vi "4 QuadEncoder PositionVelocity.vi"(0 "Quad Encoders":T1={"Encoder 0 Ch A"="Chassis1/Mod4/DI0", "Encoder 0 Ch B"="Chassis1/Mod4/DI1", "Encoder 1 Ch A"="Chassis1/Mod4/DI2", "Encoder 1 Ch B"="Chassis1/Mod4/DI3", "Encoder 2 Ch A"="Chassis1/Mod4/DI4", "Encoder 2 Ch B"="Chassis1/Mod4/DI5", "Encoder 3 Ch A"="Chassis1/Mod4/DI6", "Encoder 3 Ch B"="Chassis1/Mod4/DI7"}, 2 "Encoder Interval (uSec)":u32=1000, 4 "Position Reset":bool) -> (7 "Encoder Packets":u64[](array[numeric]))   [LabVIEW 2010]
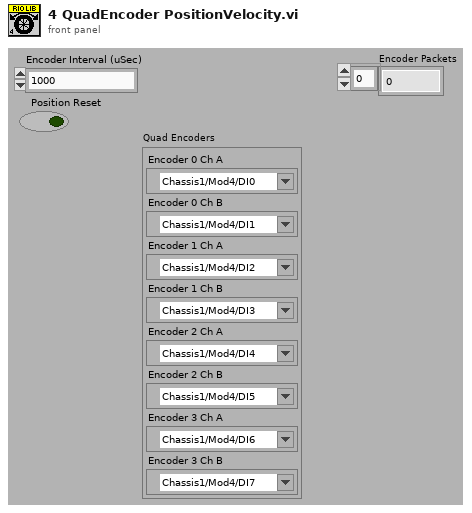
[diagram p1: front panel]
types:
  T1 = cluster{"Encoder 0 Ch A":refnum<k21>, "Encoder 0 Ch B":refnum<k21>, "Encoder 1 Ch A":refnum<k21>, "Encoder 1 Ch B":refnum<k21>, "Encoder 2 Ch A":refnum<k21>, "Encoder 2 Ch B":refnum<k21>, "Encoder 3 Ch A":refnum<k21>, "Encoder 3 Ch B":refnum<k21>}
  T2 = cluster{"Encoder 0 Ch A":refnum<k21>, "Encoder 0 Ch B":refnum<k21>}
  T3 = cluster{"Encoder 1 Ch A":refnum<k21>, "Encoder 1 Ch B":refnum<k21>}
  T4 = cluster{"Encoder 2 Ch A":refnum<k21>, "Encoder 2 Ch B":refnum<k21>}
  T5 = cluster{"Encoder 3 Ch A":refnum<k21>, "Encoder 3 Ch B":refnum<k21>}
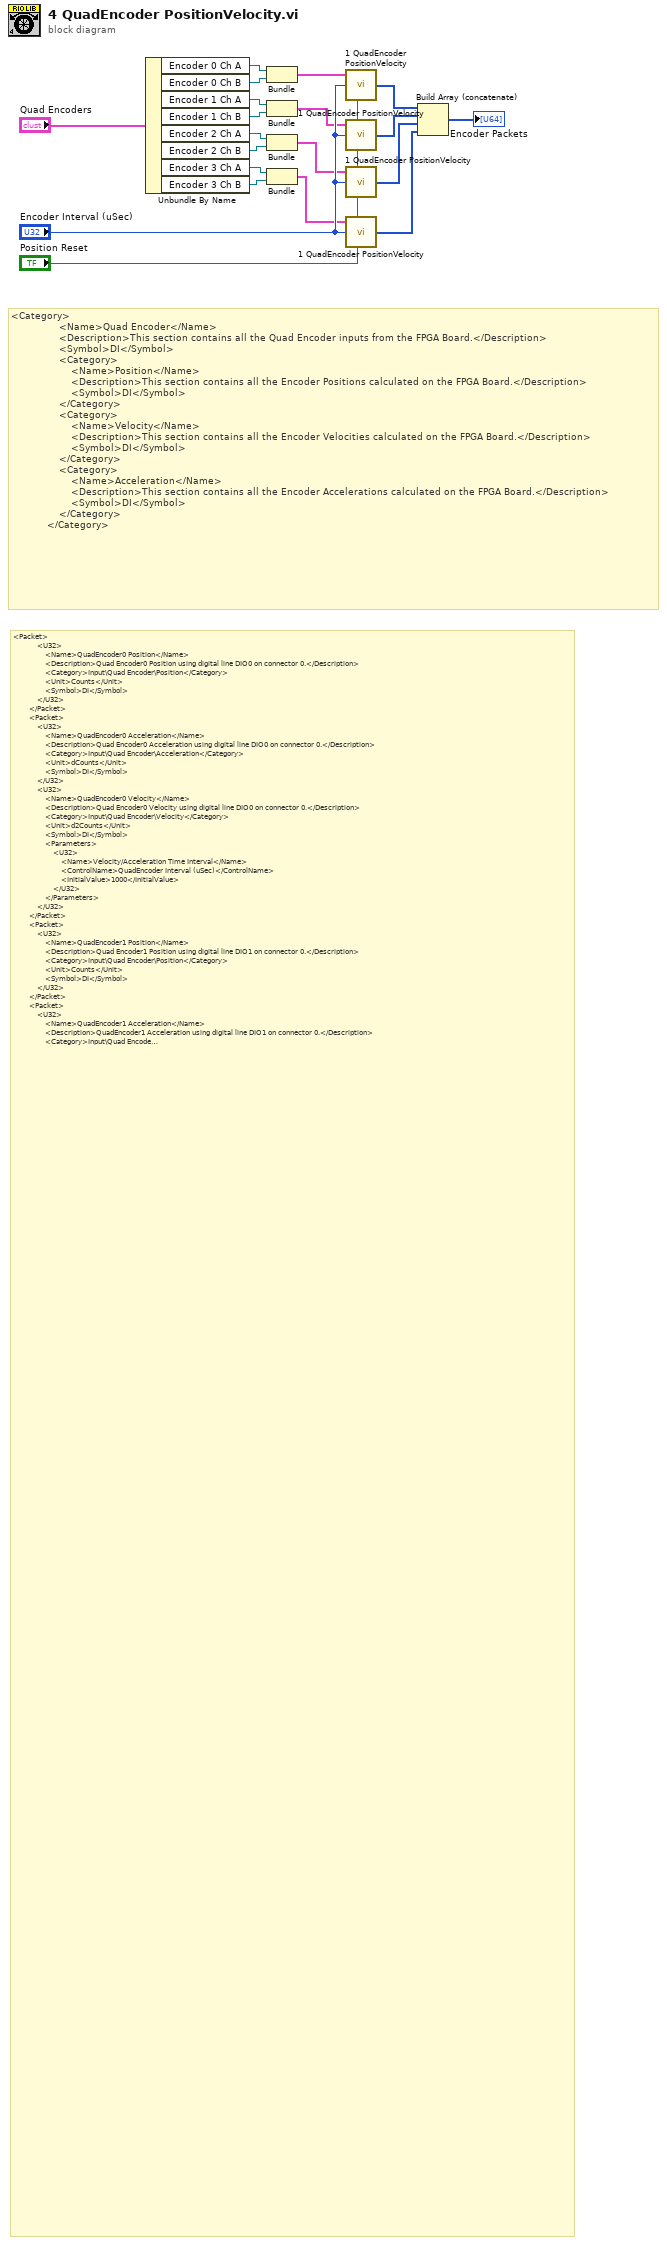
[diagram p0: block diagram]
diagram:
  # "<Category>\n                <Name>Quad Encoder</Name>\n                <Description>This section contains all the Quad Encoder inputs from the FPGA Board.</Description>\n                <Symbol>DI</Symbol>\n                <Category>\n                    <Name>Position</Name>\n                    <Description>This section contains all the Encoder Positions calculated on the FPGA Board.</Description>\n                    <Symbol>DI</Symbol>\n                </Category>\n                <Category>\n                    <Name>Velocity</Name>\n                    <Description>This section contains all the Encoder Velocities calculated on the FPGA Board.</Description>\n                    <Symbol>DI</Symbol>\n                </Category>\n                <Category>\n                    <Name>Acceleration</Name>\n                    <Description>This section contains all the Encoder Accelerations calculated on the FPGA Board.</Description>\n                    <Symbol>DI</Symbol>\n                </Category>\n            </Category>"
  # "<Packet>\n            <U32>\n                <Name>QuadEncoder0 Position</Name>\n                <Description>Quad Encoder0 Position using digital line DIO0 on connector 0.</Description>\n                <Category>Input\\Quad Encoder\\Position</Category>\n                <Unit>Counts</Unit>\n                <Symbol>DI</Symbol>\n            </U32>\n        </Packet>\n        <Packet>\n            <U32>\n                <Name>QuadEncoder0 Acceleration</Name>\n                <Description>Quad Encoder0 Acceleration using digital line DIO0 on connector 0.</Description>\n                <Category>Input\\Quad Encoder\\Acceleration</Category>\n                <Unit>dCounts</Unit>\n                <Symbol>DI</Symbol>\n            </U32>\n            <U32>\n                <Name>QuadEncoder0 Velocity</Name>\n                <Description>Quad Encoder0 Velocity using digital line DIO0 on connector 0.</Description>\n                <Category>Input\\Quad Encoder\\Velocity</Category>\n                <Unit>d2Counts</Unit>\n                <Symbol>DI</Symbol>\n                <Parameters>\n                    <U32>\n                        <Name>Velocity/Acceleration Time Interval</Name>\n                        <ControlName>QuadEncoder Interval (uSec)</ControlName>\n                        <InitialValue>1000</InitialValue>\n                    </U32>\n                </Parameters>\n            </U32>\n        </Packet>\n        <Packet>\n            <U32>\n                <Name>QuadEncoder1 Position</Name>\n                <Description>Quad Encoder1 Position using digital line DIO1 on connector 0.</Description>\n                <Category>Input\\Quad Encoder\\Position</Category>\n                <Unit>Counts</Unit>\n                <Symbol>DI</Symbol>\n            </U32>\n        </Packet>\n        <Packet>\n            <U32>\n                <Name>QuadEncoder1 Acceleration</Name>\n                <Description>QuadEncoder1 Acceleration using digital line DIO1 on connector 0.</Description>\n                <Category>Input\\Quad Encoder\\Acceleration</Category>\n                <Unit>dCounts</Unit>\n                <Symbol>DI</Symbol>\n            </U32>\n            <U32>\n                <Name>QuadEncoder1 Velocity</Name>\n                <Description>QuadEncoder1 Velocity using digital line DIO1 on connector 0.</Description>\n                <Category>Input\\Quad Encoder\\Velocity</Category>\n                <Unit>d2Counts</Unit>\n                <Symbol>DI</Symbol>\n            </U32>\n        </Packet>\n        <Packet>\n            <U32>\n                <Name>QuadEncoder2 Position</Name>\n                <Description>Quad Encoder2 Position using digital line DIO2 on connector 0.</Description>\n                <Category>Input\\Quad Encoder\\Position</Category>\n                <Unit>Counts</Unit>\n                <Symbol>DI</Symbol>\n            </U32>\n        </Packet>\n        <Packet>\n            <U32>\n                <Name>QuadEncoder2 Acceleration</Name>\n                <Description>Quad Encoder2 Acceleration using digital line DIO2 on connector 0.</Description>\n                <Category>Input\\Quad Encoder\\Acceleration</Category>\n                <Unit>dCounts</Unit>\n                <Symbol>DI</Symbol>\n            </U32>\n            <U32>\n                <Name>QuadEncoder2 Velocity</Name>\n                <Description>Quad Encoder2 Velocity using digital line DIO2 on connector 0.</Description>\n                <Category>Input\\Quad Encoder\\Velocity</Category>\n                <Unit>d2Counts</Unit>\n                <Symbol>DI</Symbol>\n            </U32>\n        </Packet>\n        <Packet>\n            <U32>\n                <Name>QuadEncoder3 Position</Name>\n                <Description>Quad Encoder3 Position using digital line DIO3 on connector 0.</Description>\n                <Category>Input\\Quad Encoder\\Position</Category>\n                <Unit>Counts</Unit>\n                <Symbol>DI</Symbol>\n            </U32>\n        </Packet>\n        <Packet>\n            <U32>\n                <Name>QuadEncoder3 Acceleration</Name>\n                <Description>QuadEncoder3 Acceleration using digital line DIO3 on connector 0.</Description>\n                <Category>Input\\Quad Encoder\\Acceleration</Category>\n                <Unit>dCounts</Unit>\n                <Symbol>DI</Symbol>\n            </U32>\n            <U32>\n                <Name>QuadEncoder3 Velocity</Name>\n                <Description>QuadEncoder3 Velocity using digital line DIO3 on connector 0.</Description>\n                <Category>Input\\Quad Encoder\\Velocity</Category>\n                <Unit>d2Counts</Unit>\n                <Symbol>DI</Symbol>\n            </U32>\n        </Packet>"
  n1 = Unbundle By Name("Quad Encoders") -> ("Encoder 0 Ch A"=w16:refnum<k21>, "Encoder 0 Ch B"=w15:refnum<k21>, "Encoder 1 Ch A"=w13:refnum<k21>, "Encoder 1 Ch B"=w12:refnum<k21>, "Encoder 2 Ch A"=w8:refnum<k21>, "Encoder 2 Ch B"=w7:refnum<k21>, "Encoder 3 Ch A"=w6:refnum<k21>, "Encoder 3 Ch B"=w5:refnum<k21>)
  n2 = Bundle("Encoder 0 Ch A"=w16, "Encoder 0 Ch B"=w15) -> (w14:T2)  [unwired: 1 in]
  n3 = Bundle("Encoder 1 Ch A"=w13, "Encoder 1 Ch B"=w12) -> (w9:T3)  [unwired: 1 in]
  n4 = Bundle("Encoder 2 Ch A"=w8, "Encoder 2 Ch B"=w7) -> (w3:T4)  [unwired: 1 in]
  n5 = Bundle("Encoder 3 Ch A"=w6, "Encoder 3 Ch B"=w5) -> (w4:T5)  [unwired: 1 in]
  n6 = call <userlib>:"1 QuadEncoder PositionVelocity.vi"("Encoder Chs"=w14, "QuadEncoder Interval (uSec)"="Encoder Interval (uSec)", "Position Reset"="Position Reset") -> ("QuadEncoder Packets"=w19:u64[])  [unwired: 6 in]
  n7 = call <userlib>:"1 QuadEncoder PositionVelocity.vi"("Encoder Chs"=w9, "QuadEncoder Interval (uSec)"="Encoder Interval (uSec)", "Position Reset"="Position Reset") -> ("QuadEncoder Packets"=w20:u64[])  [unwired: 6 in]
  n8 = call <userlib>:"1 QuadEncoder PositionVelocity.vi"("Encoder Chs"=w3, "QuadEncoder Interval (uSec)"="Encoder Interval (uSec)", "Position Reset"="Position Reset") -> ("QuadEncoder Packets"=w1:u64[])  [unwired: 6 in]
  n9 = call <userlib>:"1 QuadEncoder PositionVelocity.vi"("Encoder Chs"=w4, "QuadEncoder Interval (uSec)"="Encoder Interval (uSec)", "Position Reset"="Position Reset") -> ("QuadEncoder Packets"=w2:u64[])  [unwired: 6 in]
  n10 = Build Array (concatenate)(w19, w20, w1, w2) -> (→"Encoder Packets":u64[])
